vi "Create Request.vi"(8 "error in (no error)":errorcluster, 9 "params":variant, 10 "method":string, 11 "Request":refnum<class "Request.lvclass">) -> (0 "error out":errorcluster, 2 "JSON Request":string, 3 "Request out":refnum<class "Request.lvclass">)   [LabVIEW 2019, in "Request.lvclass"]
uses:
  Request.lvclass
  typedefs/JSON-RPC-Request Object--Cluster.ctl
  Request.lvclass/Request.ctl
  lv-venv/lv.lib/vi.lib/addons/_JKI.lib/Serialization/JSON/JKI JSON Serialization.lvlib
  JSON-RPC.lvclass
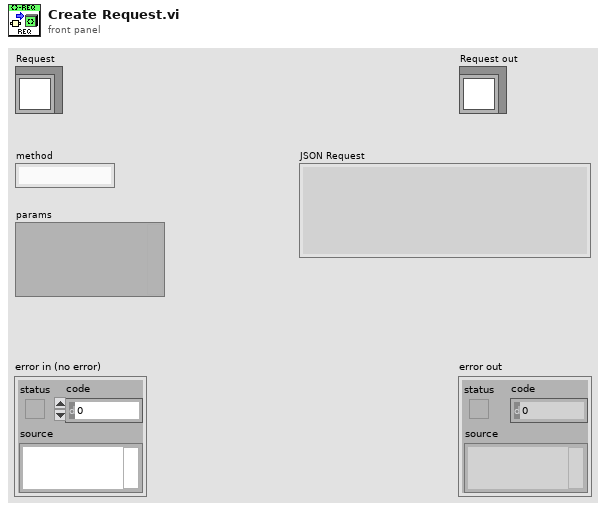
[diagram p1: front panel]
types:
  T1 = typedef "JSON-RPC.lvclass/JSON-RPC-Request Object--Cluster.ctl" = cluster{"jsonrpc":string, "method":string, "params":variant, "id":string}
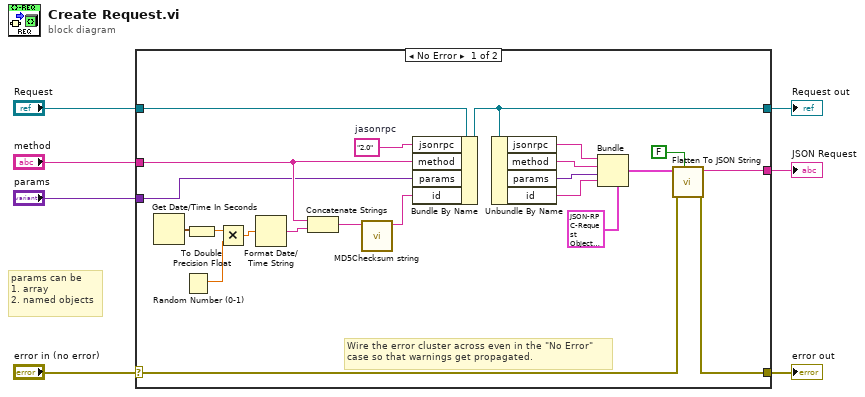
[diagram p0: block diagram]
diagram:
  # "params can be\n1. array\n2. named objects"
  n1 = case shown="No Error" "error in (no error)" {
    selector: "error in (no error)" -> [w25 w31]
    tunnel: [w24 w31] -> w6
    tunnel: [w17 w30] -> w5
    tunnel: "method" -> [w21 _]
    tunnel: "params" -> [w20 _]
    tunnel: "Request" -> [w27 w30]
    tunnel: [w23 _] -> w1
    frame No Error {
      w22 = "2.0"  # jasonrpc
      # "Wire the error cluster across even in the \"No Error\"\ncase so that warnings get propagated."
      n2 = Get Date/Time In Seconds() -> (seconds since 1Jan1904=w11:timestamp)
      n3 = Random Number (0-1)() -> (number: 0 to 1=w8:dbl)
      n4 = To Double Precision Float(number=w11) -> (double precision float=w10:dbl)
      n5 = Multiply(x=w10, y=w8) -> (x*y=w9:dbl)
      n6 = Format Date/Time String(seconds (now)=w9) -> (date/time string=w28:string)  [unwired: 2 in]
      n7 = Concatenate Strings(w21, w28) -> (w29:string)
      n8 = call <vilib>:"MD5Checksum string.vi"("Message String"=w29) -> ("MD5 message-digest"=w18:string)  [unwired: 10 in]
      n9 = Bundle By Name(cluster=w27, "jsonrpc"=w22, "method"=w21, "params"=w20, "id"=w18) -> (w17:refnum<class "Request.lvclass">)
      n10 = Unbundle By Name(w17) -> ("jsonrpc"=w16:string, "method"=w13:string, "params"=w14:variant, "id"=w15:string)
      n11 = Bundle(cluster=T1 {"jsonrpc"="", "method"="", "params"=variant, "id"=""} ("request"), "jsonrpc"=w16, "method"=w13, "params"=w14, "id"=w15) -> (w19:T1)
      n12 = call "Flatten To JSON String.vi"("Multiline (T)"=FALSE, "error in (no error)"=w25, "Variant"=w19) -> ("error out"=w24:errorcluster, "JSON String"=w23:string)  [unwired: 7 in]
    }
    frame Error {
    }
  }
  "error out" <- w6
  "Request out" <- w5
  "JSON Request" <- w1
